vi "Helper - Load Image Descriptor.vi"(11 "Image Descriptor File Path":path) -> (3 "Image Descriptor Typedef out":T1)   [LabVIEW 2011]
doc: "Opens an image descriptor from a file. Image descriptors are used for converting between image coordinates and UTM."
uses:
  0-OCU/0 Code/mission input/0-Image Descriptor.ctl
  2 Typedefs/UTM Location.ctl
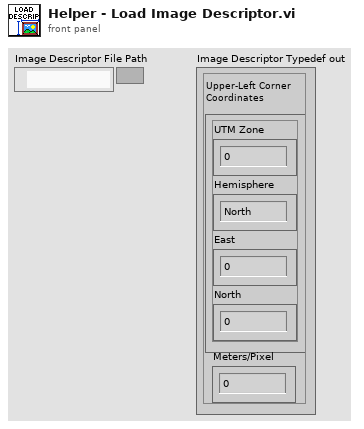
[diagram p1: front panel]
types:
  T1 = typedef "0-Image Descriptor.ctl" = cluster{"Upper-Left Corner Coordinates":T2, "Meters/Pixel":dbl}
  T2 = typedef "UTM Location.ctl" = cluster{"UTM Zone":dbl, "Hemisphere":enum16{"North", "South"}, "East":dbl, "North":dbl}
  T3 = enum16{"open", "replace", "create", "open or create", "replace or create", "replace or create with confirmation"}
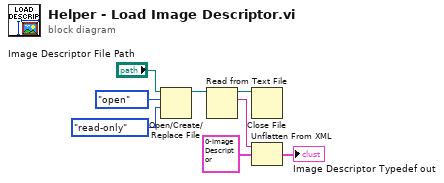
[diagram p0: block diagram]
diagram:
  n1 = Open/Create/Replace File(file path (use dialog)="Image Descriptor File Path", operation (0:open)=T3."open", access (0:read/write)=enum16{"read/write", "read-only", "write-only"}."read-only") -> (refnum out=w4:refnum<file>)  [unwired: 1 in, 4 out]
  n2 = Read from Text File(file (use dialog)=w4) -> (refnum out=w5:refnum<file>, text=w7:string)  [unwired: 1 in, 4 out]
  n3 = Close File(refnum=w5) -> ()  [unwired: 1 in, 2 out]
  n4 = Unflatten From XML(xml string=w7, type=T1 {"Upper-Left Corner Coordinates"={"UTM Zone"=0.0, "Hemisphere"=enum."North", "East"=0.0, "North"=0.0}, "Meters/Pixel"=42.294203} ("Image Descriptor Typedef in")) -> (value=→"Image Descriptor Typedef out":T1)  [unwired: 1 in, 1 out]
